vi "autonSample.vi"(0 "Auton Array":dbl[][](array[numeric]), 5 "MeasuredHeading":dbl, 9 "EncoderDistance":dbl) -> (4 "Left Drive":dbl(knob) scale=-1.0..1.0, 6 "Right Drive":dbl(knob) scale=-1.0..1.0, 10 "Turret Rotation":dbl, 14 "Feeder motor":dbl, 15 "Shooter motor output":dbl)   [LabVIEW 2011]
uses:
  Robot Global Data.vi
  <vilib>/addons/control/pid/pid.llb/PID (DBL).vi
  <vilib>/addons/control/pid/NI_PID_pid.lvlib
panel:
  out "Tzero":i64
  out "AccumDist":dbl
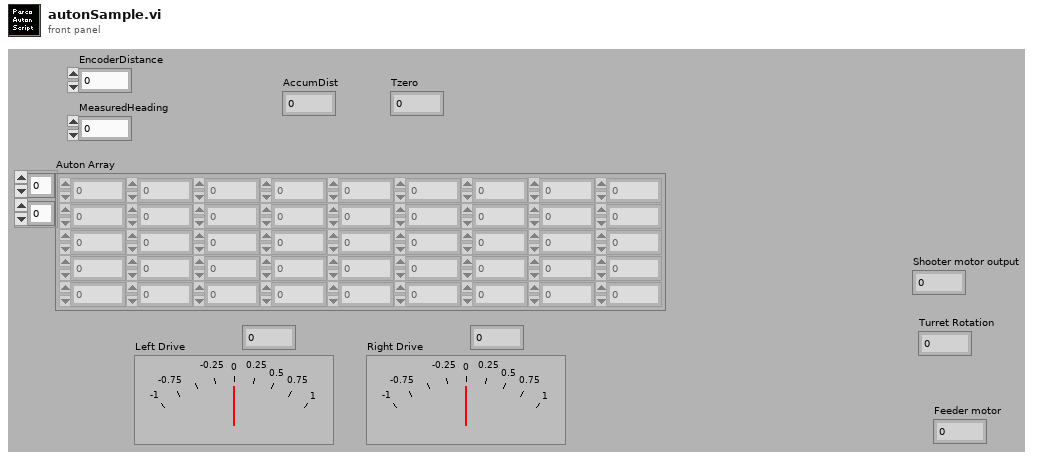
[diagram p1: front panel]
types:
  T1 = cluster{"proportional gain (Kc)":dbl, "integral time (Ti, min)":dbl, "derivative time (Td, min)":dbl}
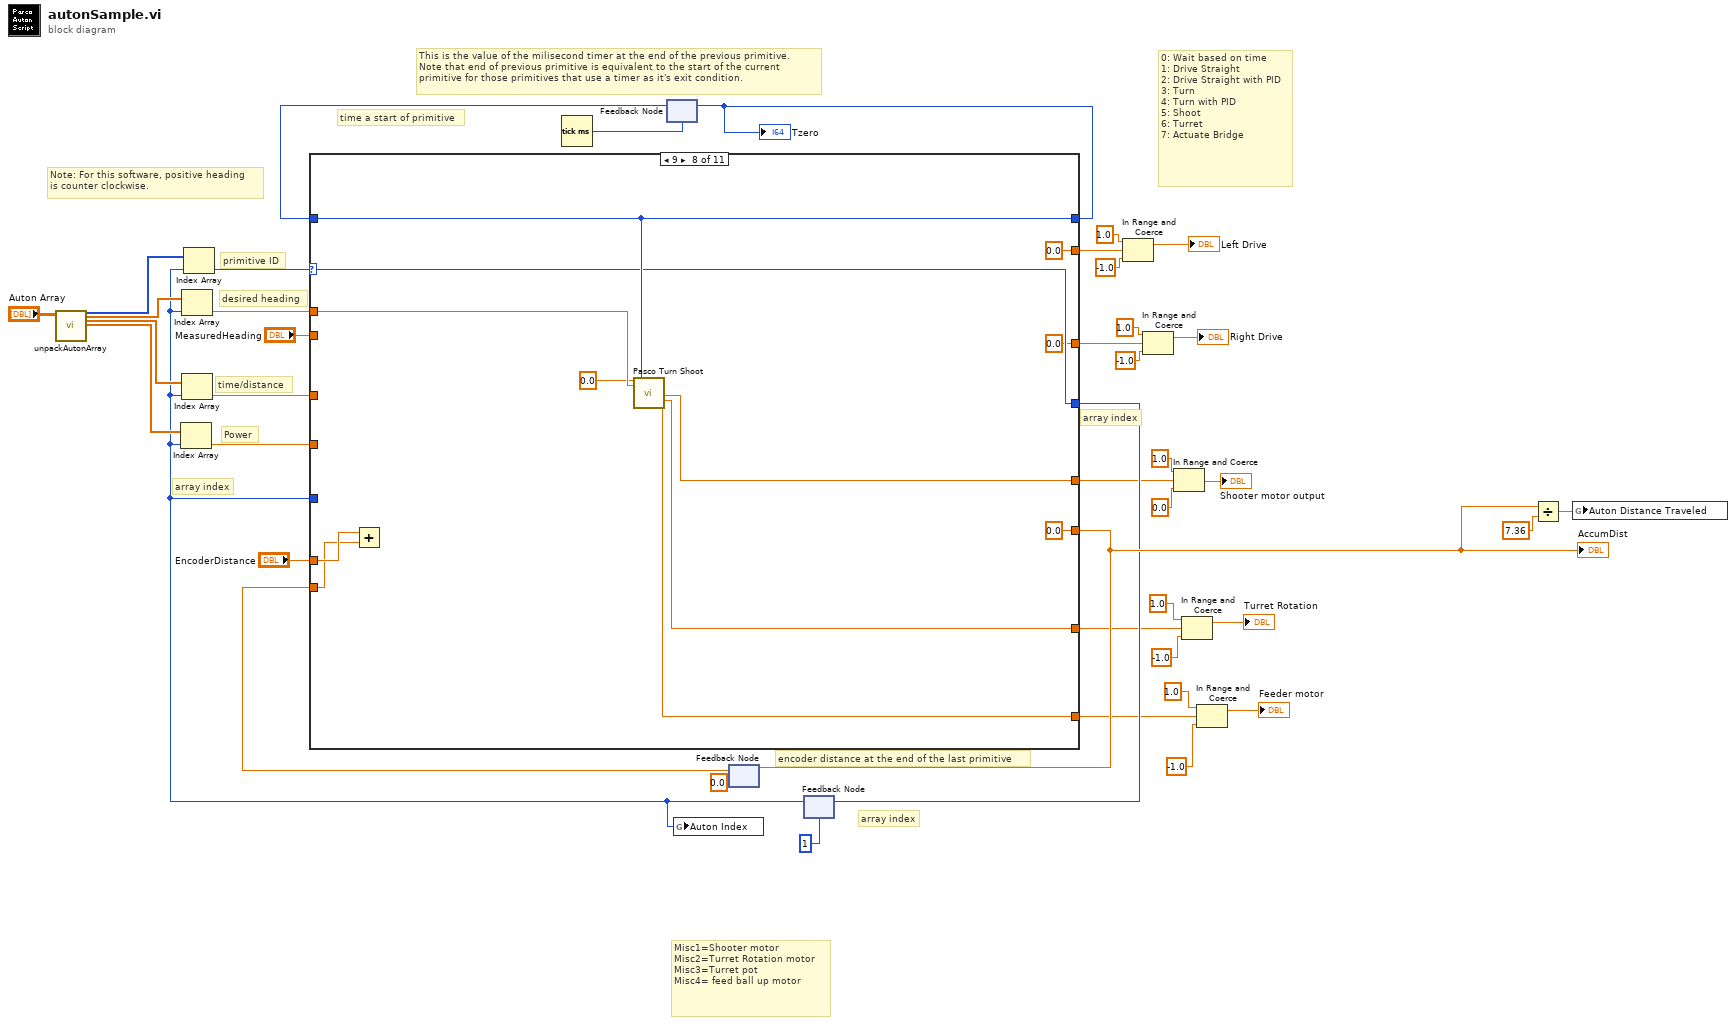
[diagram p0: block diagram]
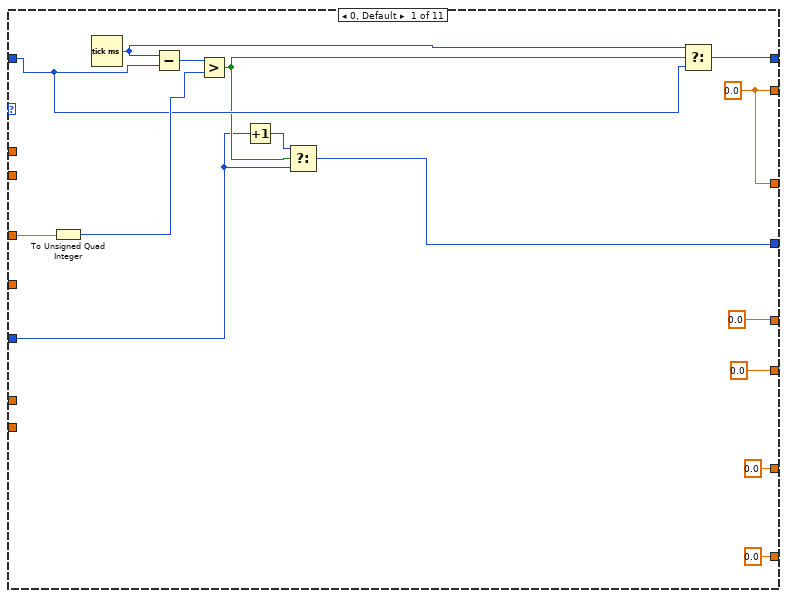
[diagram p2: hidden frame]
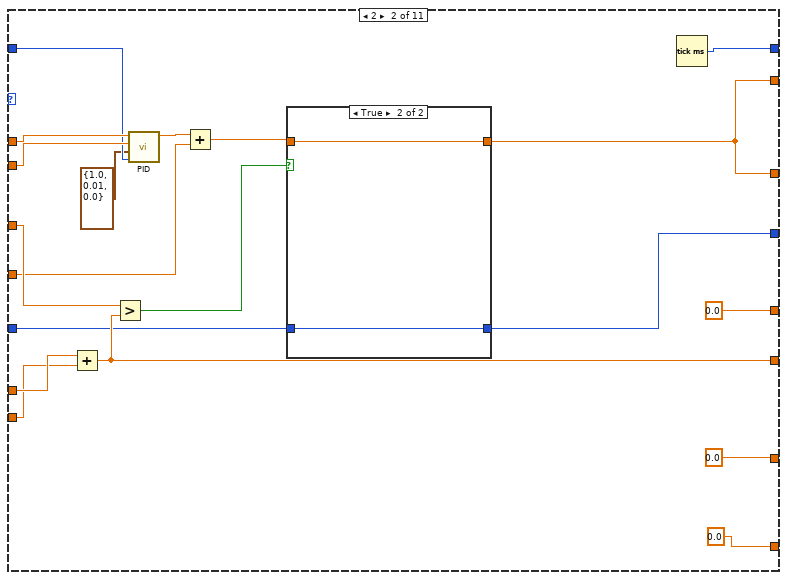
[diagram p3: hidden frame]
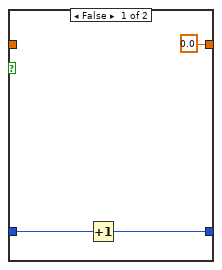
[diagram p4: hidden frame]
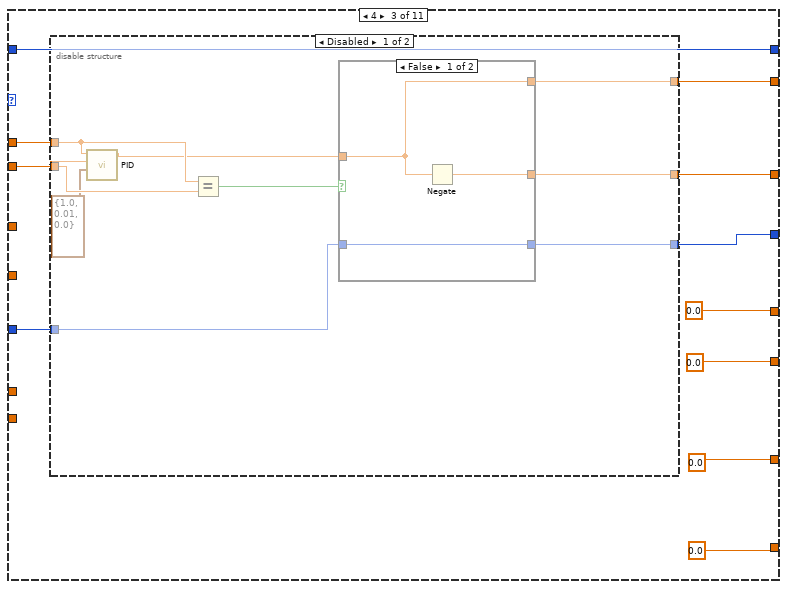
[diagram p5: hidden frame]
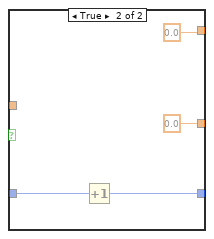
[diagram p6: hidden frame]
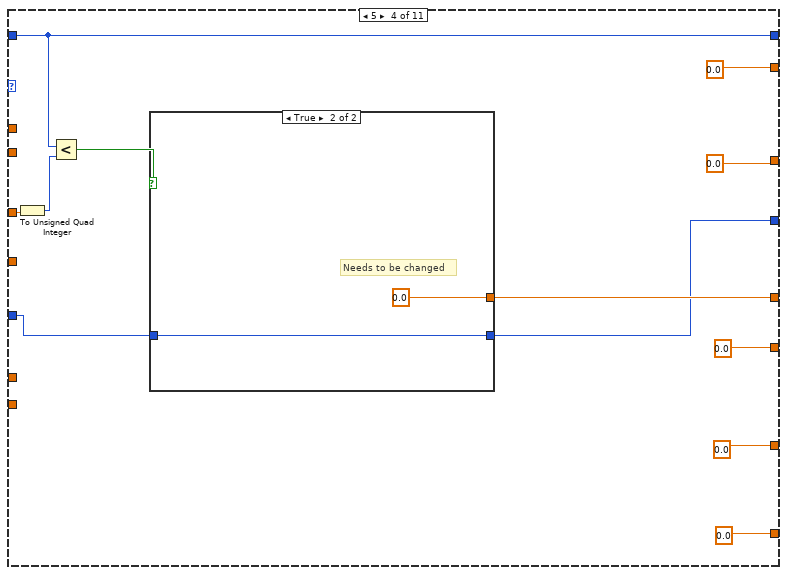
[diagram p8: hidden frame]
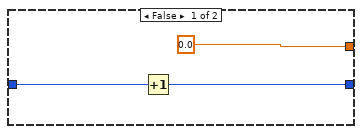
[diagram p9: hidden frame]
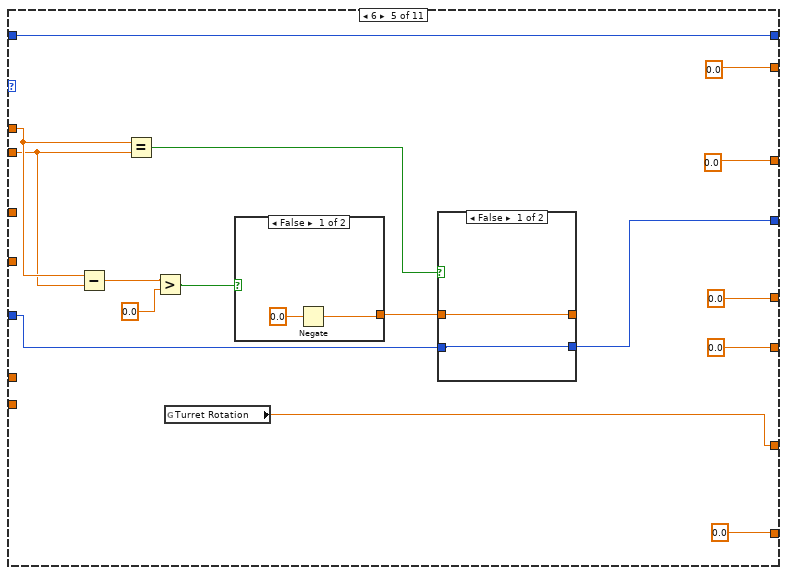
[diagram p10: hidden frame]
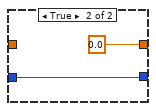
[diagram p11: hidden frame]
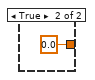
[diagram p12: hidden frame]
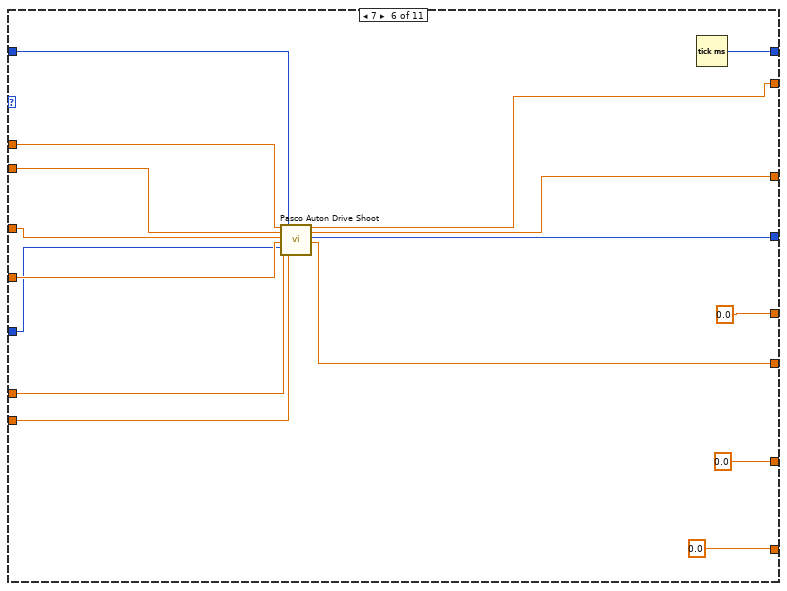
[diagram p13: hidden frame]
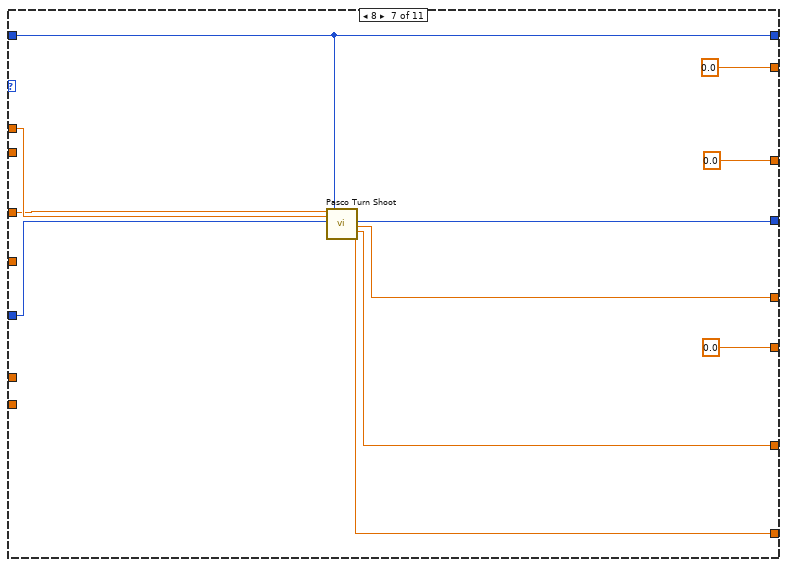
[diagram p14: hidden frame]
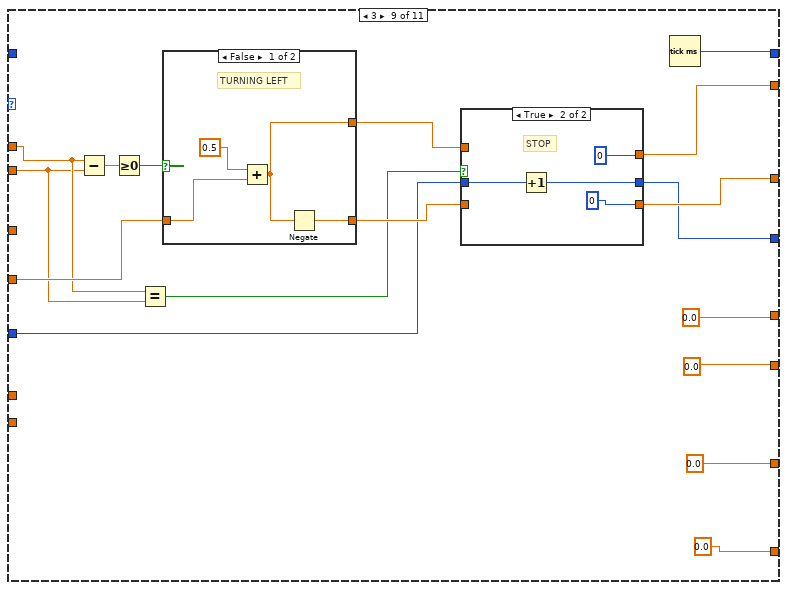
[diagram p15: hidden frame]
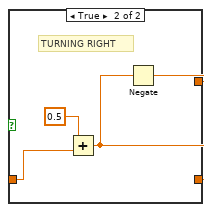
[diagram p17: hidden frame]
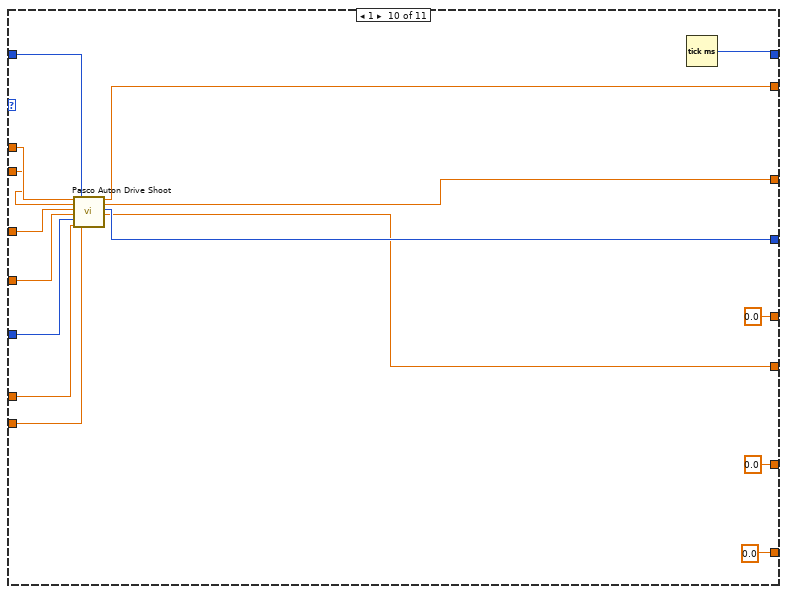
[diagram p18: hidden frame]
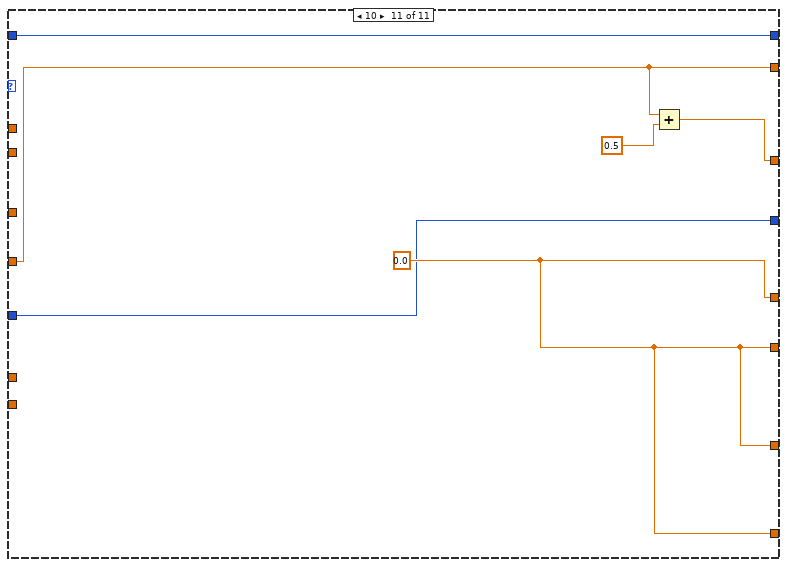
[diagram p19: hidden frame]
diagram:
  # "Misc1=Shooter motor\nMisc2=Turret Rotation motor\nMisc3=Turret pot\nMisc4= feed ball up motor"
  # "0: Wait based on time\n1: Drive Straight\n2: Drive Straight with PID\n3: Turn\n4: Turn with PID\n5: Shoot\n6: Turret\n7: Actuate Bridge"
  # "encoder distance at the end of the last primitive"
  # "Note: For this software, positive heading\nis counter clockwise."
  # "time a start of primitive"
  # "array index"
  # "array index"
  # "This is the value of the milisecond timer at the end of the previous primitive.\nNote that end of previous primitive is equivalent to the start of the current\nprimitive for those primitives that use a timer as it's exit condition."
  # "Power"
  # "array index"
  # "desired heading"
  # "primitive ID"
  # "time/distance"
  n1 = call "unpackAutonArray.vi"("all rows"="Auton Array") -> ("Primitive"=w41:i16[], "Heading"=w23:dbl[], "Distance/Time"=w24:dbl[], "Power"=w21:dbl[])  [unwired: 1 in, 22 out]
  n2 = Tick Count (ms)() -> (millisecond timer value=w35:u32)
  n3 = feedback #1(w35) -> (w39:u32)
  n4 = feedback #2(0.0 ("EncoderDistance")) -> (w20:dbl)
  n5 = feedback #3(1) -> (w2:i32)
  n6 = Index Array(array=w21, index=w2) -> (element=w37:dbl)
  n7 = Index Array(array=w23, index=w2) -> (element=w22:dbl)
  n8 = Index Array(array=w24, index=w2) -> (element=w38:dbl)
  n9 = Index Array(array=w41, index=w2) -> (element=w40:i16)
  n10 = case shown="9" w40 {
    selector: w40 -> [_ _ _ _ _ _ _ w178 _ _ _]
    tunnel: [w45 w69 w86 w115 w137 w149 w172 w178 w193 w222 w240] -> w15
    tunnel: w2 -> [w46 w70 w85 w116 w138 w156 w175 _ w192 w228 w240]
    tunnel: [w57 w76 w92 w110 w136 w162 w173 w182 w199 w234 w239] -> w25
    tunnel: w39 -> [w53 w63 w92 w110 w136 w153 w173 w182 _ w225 w239]
    tunnel: w38 -> [w55 w72 _ w120 _ w158 w169 _ _ w230 _]
    tunnel: w22 -> [_ w64 w82 _ w141 w160 w174 w185 w201 w232 _]
    tunnel: [w44 w71 w87 0.0 0.0 w152 0.0 0.0 ("Numeric") w195 w224 w237] -> w33
    tunnel: [w44 w71 w88 0.0 0.0 w151 0.0 0.0 ("Right Drive") w198 w223 w236] -> w26
    tunnel: w37 -> [_ w60 _ _ _ w157 _ _ w203 w229 w237]
    tunnel: "EncoderDistance" -> [_ w75 _ _ _ w154 _ w187 _ w227 _]
    tunnel: "MeasuredHeading" -> [_ w65 w83 _ w127 w159 _ _ w200 w231 _]
    tunnel: [0.0 ("Encoder total") w73 0.0 0.0 0.0 w150 0.0 0.0 ("Encoder total") 0.0 w221 w241] -> w17
    tunnel: w20 -> [_ w74 _ _ _ w155 _ w186 _ w226 _]
    tunnel: [0.0 ("Misc1  OUT") 0.0 0.0 w117 0.0 0.0 ("Misc1  OUT") w171 w184 0.0 0.0 ("Misc1  OUT") w241] -> w11
    tunnel: [0.0 ("Misc2 OUT") 0.0 0.0 0.0 w126 0.0 ("Misc1  OUT") w170 w183 0.0 0.0 ("Misc2 OUT") w241] -> w7
    tunnel: [0.0 ("Misc4 OUT") 0.0 0.0 0.0 0.0 0.0 w165 w180 0.0 0.0 w241] -> w3
    frame 0, Default {
      w44 = 0.0 ("Numeric")
      n11 = To Unsigned Quad Integer(1:w55) -> (0:w54:u64)
      n12 = Tick Count (ms)() -> (millisecond timer value=w52:u32)
      n13 = Subtract(x=w52, y=w53) -> (x-y=w56:u32)
      n14 = Greater?(x=w56, y=w54) -> (0:w48:bool)
      n15 = Increment(x=w46) -> (x+1=w47:i32)
      n16 = Select(t=w47, s=w48, f=w46) -> (s? t:f=w45:i32)
      n17 = Select(t=w52, s=w48, f=w53) -> (s? t:f=w57:u32)
    }
    frame 2 {
      n18 = Add(x=w75, y=w74) -> (x+y=w73:dbl)
      n19 = Greater?(x=w72, y=w73) -> (0:w62:bool)
      n20 = call-poly <vilib>:"PID.vi"("dt (s)"=w63, "PID gains"=T1 {"proportional gain (Kc)"=1.0, "integral time (Ti, min)"=0.01, "derivative time (Td, min)"=0.0}, "process variable"=w65, "setpoint"=w64) -> ("output"=w59:dbl)  [unwired: 6 in, 1 out]
      n21 = Add(x=w59, y=w60) -> (x+y=w58:dbl)
      n22 = case shown="True" w62 {
        tunnel: [0.0 w81] -> w71
        tunnel: w58 -> [_ w81]
        tunnel: w70 -> [w79 w80]
        tunnel: [w78 w80] -> w69
        frame False {
          n23 = Increment(x=w79) -> (x+1=w78:i32)
        }
        frame True {
        }
      }
      n24 = Tick Count (ms)() -> (millisecond timer value=w76:u32)
    }
    frame 4 {
      n25 = disable-structure shown="Disabled" {
        disable-tunnel: [w101 _] -> w88
        disable-tunnel: [w100 _] -> w87
        disable-tunnel: [w99 _] -> w86
        disable-tunnel: w85 -> [w98 _]
        disable-tunnel: w83 -> [w96 _]
        disable-tunnel: w82 -> [w95 _]
        frame Disabled {
          n26 = call-poly <vilib>:"PID.vi"("PID gains"=T1 {"proportional gain (Kc)"=1.0, "integral time (Ti, min)"=0.01, "derivative time (Td, min)"=0.0}, "process variable"=w96, "setpoint"=w95) -> ("output"=w94:dbl)  [unwired: 7 in, 1 out]
          n27 = Equal?(x=w95, y=w96) -> (x = y?=w97:bool)
          n28 = case shown="False" w97 {
            tunnel: w94 -> [w103 _]
            tunnel: [w104 0.0] -> w101
            tunnel: [w103 0.0] -> w100
            tunnel: [w102 w107] -> w99
            tunnel: w98 -> [w102 w108]
            frame False {
              n29 = Negate(x=w103) -> (-x=w104:dbl)
            }
            frame True {
              n30 = Increment(x=w108) -> (x+1=w107:i32)
            }
          }
        }
        frame Enabled {
        }
      }
    }
    frame 5 {
      n31 = To Unsigned Quad Integer(1:w120) -> (0:w118:u64)
      n32 = Less?(x=w110, y=w118) -> (x < y?=w119:bool)
      n33 = case shown="True" w119 {
        tunnel: [0.0 0.0] -> w117
        tunnel: w116 -> [w122 w125]
        tunnel: [w121 w125] -> w115
        frame False {
          n34 = Increment(x=w122) -> (x+1=w121:i32)
        }
        frame True {
          # "Needs to be changed"
        }
      }
    }
    frame 6 {
      n35 = Subtract(x=w141, y=w127) -> (x-y=w129:dbl)
      n36 = Equal?(x=w141, y=w127) -> (x = y?=w140:bool)
      n37 = Greater?(x=w129, y=0.0) -> (0:w130:bool)
      n38 = global read "Robot Global Data.vi" "Turret Rotation"() -> (w126:dbl)
      n39 = case shown="False" w130 {
        tunnel: [w147 0.0] -> w139
        frame False {
          n40 = Negate(x=0.0) -> (-x=w147:dbl)
        }
        frame True {
        }
      }
      n41 = case shown="False" w140 {
        tunnel: [w143 0.0] -> _
        tunnel: w139 -> [w143 _]
        tunnel: w138 -> [w142 w145]
        tunnel: [w142 w145] -> w137
        frame False {
        }
        frame True {
        }
      }
    }
    frame 7 {
      n42 = call "Pasco Auton Drive Shoot.vi"("Desired Heading"=w160, "Actual Heading"=w159, "time/distance"=w158, "Power"=w157, "Array"=w156, "Encoder total"=w154, "Time"=w153, "Encoder Return"=w155) -> ("Left Drive"=w152:dbl, "Right Drive"=w151:dbl, "Array Out"=w149:i32, "Encoder total"=w150:dbl)  [unwired: 8 in]
      n43 = Tick Count (ms)() -> (millisecond timer value=w162:u32)
    }
    frame 8 {
      n44 = call "Pasco Turn Shoot.vi"("time/distance"=w169, "desired heading"=w174, "array index"=w175, "primitive time"=w173) -> ("array index"=w172:i32, "Misc1  OUT"=w171:dbl, "Misc2 OUT"=w170:dbl, "Misc4 OUT"=w165:dbl)  [unwired: 12 in]
    }
    frame 9 {
      n45 = Add(x=w187, y=w186) -> ()  [unwired: 1 out]
      n46 = call "Pasco Turn Shoot.vi"("time/distance"=0.0, "desired heading"=w185, "primitive time"=w182) -> ("Misc1  OUT"=w184:dbl, "Misc2 OUT"=w183:dbl, "Misc4 OUT"=w180:dbl)  [unwired: 13 in, 1 out]
    }
    frame 3 {
      n47 = Subtract(x=w201, y=w200) -> (x-y=w204:dbl)
      n48 = Greater Or Equal To 0?(x=w204) -> (x >= 0?=w202:bool)
      n49 = Equal?(x=w201, y=w200) -> (x = y?=w194:bool)
      n50 = case shown="False" w202 {
        tunnel: w203 -> [w214 w216]
        tunnel: [w212 w218] -> w196
        tunnel: [w213 w217] -> w197
        frame False {
          # "TURNING LEFT"
          n51 = Add(x=0.5, y=w214) -> (x+y=w212:dbl)
          n52 = Negate(x=w212) -> (-x=w213:dbl)
        }
        frame True {
          # "TURNING RIGHT"
          n53 = Add(x=0.5, y=w216) -> (x+y=w217:dbl)
          n54 = Negate(x=w217) -> (-x=w218:dbl)
        }
      }
      n55 = case shown="True" w194 {
        tunnel: w192 -> [w207 w211]
        tunnel: [w207 w210] -> w193
        tunnel: [w206 0] -> w198
        tunnel: w197 -> [w206 _]
        tunnel: [w205 0] -> w195
        tunnel: w196 -> [w205 _]
        frame False {
          # "DRIVE"
        }
        frame True {
          # "STOP"
          n56 = Increment(x=w211) -> (x+1=w210:i32)
        }
      }
      n57 = Tick Count (ms)() -> (millisecond timer value=w199:u32)
    }
    frame 1 {
      n58 = call "Pasco Auton Drive Shoot.vi"("Desired Heading"=w232, "Actual Heading"=w231, "time/distance"=w230, "Power"=w229, "Array"=w228, "Encoder total"=w227, "Time"=w225, "Encoder Return"=w226) -> ("Left Drive"=w224:dbl, "Right Drive"=w223:dbl, "Array Out"=w222:i32, "Encoder total"=w221:dbl)  [unwired: 8 in]
      n59 = Tick Count (ms)() -> (millisecond timer value=w234:u32)
    }
    frame 10 {
      w241 = 0.0
      n60 = Add(x=w237, y=0.5 ("x+y")) -> (x+y=w236:dbl)
    }
  }
  "AccumDist" <- w17
  "Tzero" <- w25
  n61 = feedback-in #1(w25) -> ()
  n62 = global write "Robot Global Data.vi" "Auton Index"(w2) -> ()
  n63 = feedback-in #2(w17) -> ()
  n64 = feedback-in #3(w15) -> ()
  n65 = In Range and Coerce(upper limit=1.0, x=w33, lower limit=-1.0) -> (coerced(x)=→"Left Drive":dbl)  [unwired: 1 out]
  n66 = In Range and Coerce(upper limit=1.0, x=w26, lower limit=-1.0) -> (coerced(x)=→"Right Drive":dbl)  [unwired: 1 out]
  n67 = In Range and Coerce(upper limit=1.0, x=w11, lower limit=0.0) -> (coerced(x)=→"Shooter motor output":dbl)  [unwired: 1 out]
  n68 = In Range and Coerce(upper limit=1.0, x=w7, lower limit=-1.0) -> (coerced(x)=→"Turret Rotation":dbl)  [unwired: 1 out]
  n69 = In Range and Coerce(upper limit=1.0, x=w3, lower limit=-1.0) -> (coerced(x)=→"Feeder motor":dbl)  [unwired: 1 out]
  n70 = Divide(x=w17, y=7.36) -> (x/y=w1:dbl)
  n71 = global write "Robot Global Data.vi" "Auton Distance Traveled"(w1) -> ()
